vi "Motor_Controller_Tune.vi"(4 "Friction Compensation(F)":bool, 6 "Reinitialize? (F)":bool, 7 "Softload? (T)":bool=TRUE, 8 "error in (no error)":errorcluster, 9 "Mode":T2, 10 "CableTensionRef(N)":dbl[](array[numeric]), 11 "Motor in":refnum<class "MotorControl.lvclass">) -> (0 "error out":errorcluster, 1 "Detailed Voltage":T1, 2 "VoltageCommand":dbl[](array[numeric]) format="%.2f", 3 "Motor out":refnum<class "MotorControl.lvclass">, 5 "PID Gain Idx":i32[](array[numeric]))   [LabVIEW 2015, in "MotorControl.lvclass"]
uses:
  MotorControl.lvclass
  TypeDef/MotorMode.ctl
  MotorControl.lvclass/MotorControl.ctl
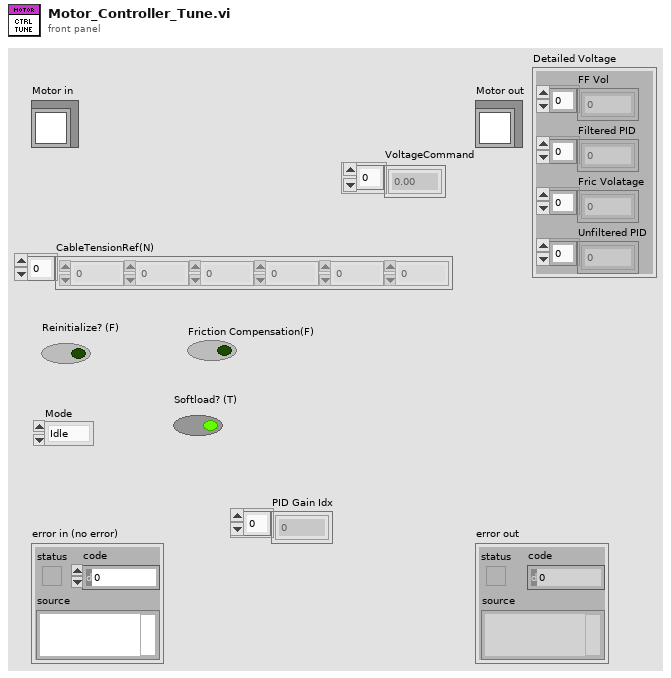
[diagram p1: front panel]
types:
  T1 = cluster{"FF Vol":dbl[], "Filtered PID":dbl[], "Fric Volatage":dbl[], "Unfiltered PID":dbl[]}
  T2 = typedef "MotorControl.lvclass/MotorMode.ctl" = enum16{"Idle", "FF", "PID"}
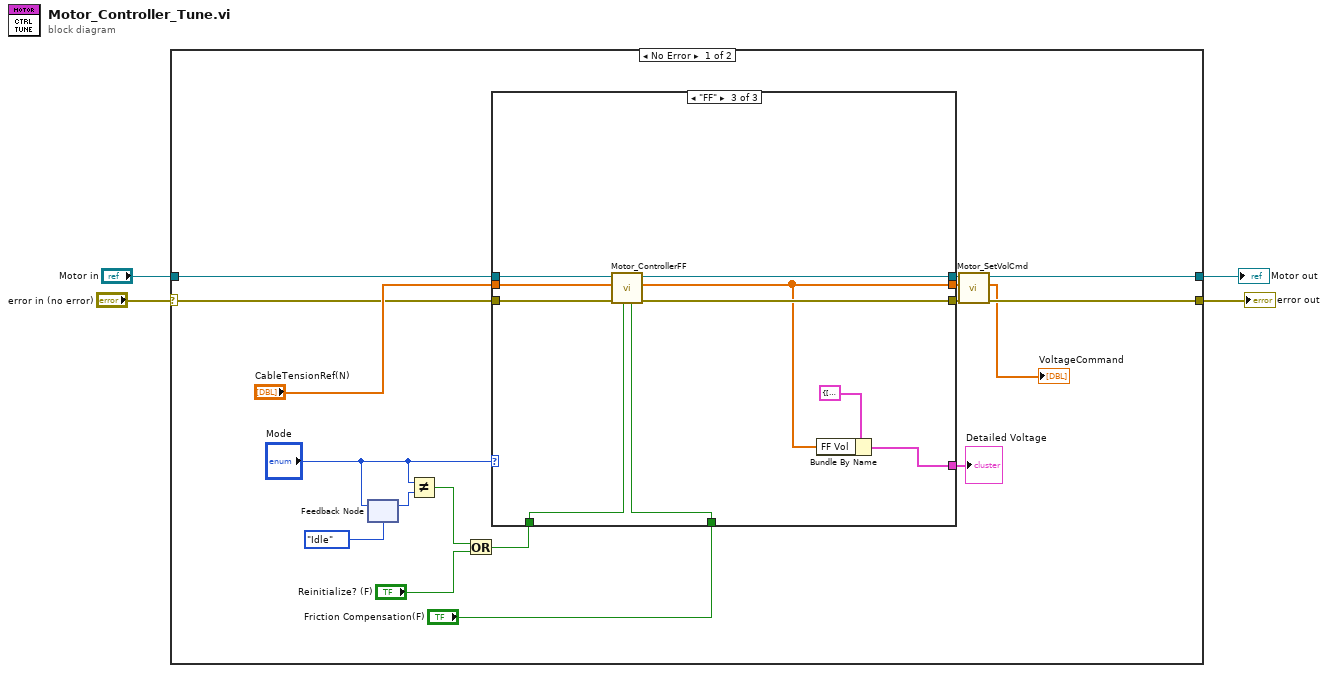
[diagram p0: block diagram]
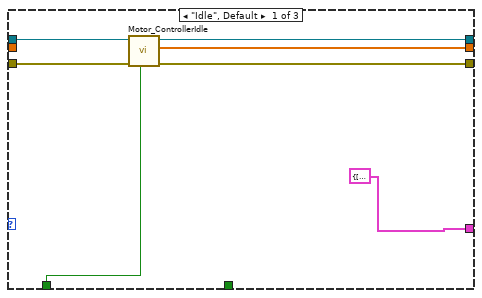
[diagram p2: hidden frame]
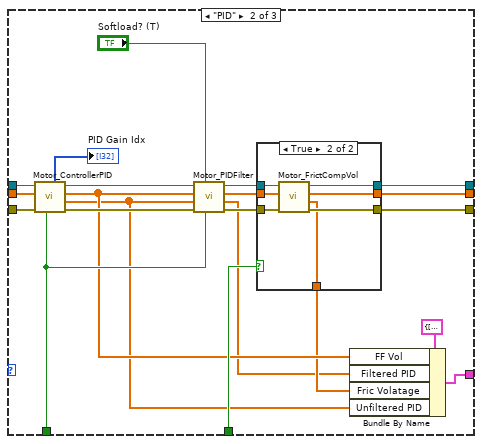
[diagram p3: hidden frame]
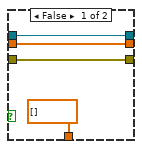
[diagram p4: hidden frame]
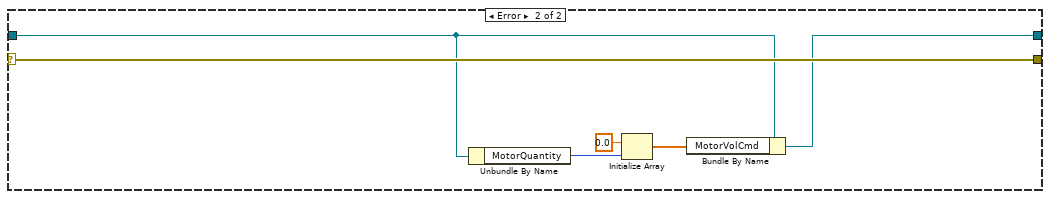
[diagram p5: hidden frame]
diagram:
  n1 = case shown="No Error" "error in (no error)" {
    selector: "error in (no error)" -> [w20 w76]
    tunnel: [w9 w76] -> w3
    tunnel: [w11 w71] -> w1
    tunnel: "Motor in" -> [w19 w72]
    frame No Error {
      n2 = feedback-in #1("Mode") -> ()
      n3 = feedback #1(MotorMode."Idle" ("Mode")) -> (w17:T2)
      n4 = Not Equal?(x="Mode", y=w17) -> (x != y?=w15:bool)
      n5 = Or(x=w15, y="Reinitialize? (F)") -> (x .or. y?=w13:bool)
      n6 = case shown="\"FF\"" "Mode" {
        tunnel: "CableTensionRef(N)" -> [_ w47 w70]
        tunnel: w20 -> [w28 w49 w69]
        tunnel: w19 -> [w27 w48 w68]
        tunnel: w13 -> [w24 w43 w67]
        tunnel: [w25 w39 w66] -> w10
        tunnel: [w26 w40 w65] -> w12
        tunnel: [w23 w36 w63] -> w7
        tunnel: "Friction Compensation(F)" -> [_ w38 w64]
        tunnel: [T1 {"FF Vol"=[], "Filtered PID"=[], "Fric Volatage"=[], "Unfiltered PID"=[]} ("Detailed Voltage") w31 w61] -> w5
        frame "Idle", Default {
          n7 = call "Motor_ControllerIdle.vi"("Reinitialize"=w24, "error in (no error)"=w28, "Motor Control in"=w27) -> ("error out"=w25:errorcluster, "VoltageCommand"=w23:dbl[], "Motor Control out"=w26:refnum<class "MotorControl.lvclass">)  [unwired: 6 in]
        }
        frame "PID" {
          n8 = call "Motor_ControllerPID.vi"("Reinitialize? (F)"=w43, "error in (no error)"=w49, "CableTensionRef(N)"=w47, "Motor in"=w48) -> ("error out"=w45:errorcluster, "PID cmd"=w29:dbl[], "FF cmd"=w34:dbl[], "Motor out"=w46:refnum<class "MotorControl.lvclass">, "PID Gain Idx"=→"PID Gain Idx":i32[])  [unwired: 2 in, 1 out]
          n9 = call "Motor_PIDFilter.vi"("Initialize (F)"=w43, "Softload? (T)"="Softload? (T)", "error in (no error)"=w45, "PID cmd in"=w29, "FF cmd in"=w34, "Motors_New in"=w46) -> ("error out"=w42:errorcluster, "Filtered PID"=w32:dbl[], "Filtered PID + FF"=w37:dbl[], "Motors_New out"=w41:refnum<class "MotorControl.lvclass">)  [unwired: 2 in]
          n10 = case shown="True" w38 {
            tunnel: w42 -> [w52 w60]
            tunnel: w41 -> [w53 w59]
            tunnel: [w53 w58] -> w40
            tunnel: [w52 w57] -> w39
            tunnel: [dbl[] [] ("Fric Volatage") w54] -> w33
            tunnel: w37 -> [w50 w56]
            tunnel: [w50 w55] -> w36
            frame False {
            }
            frame True {
              n11 = call-dynamic "Motor_FrictCompVol.vi"("error in (no error)"=w60, "Input Vol"=w56, "Motor in"=w59) -> ("error out"=w57:errorcluster, "Fric Volatage"=w54:dbl[], "Fric Vol + Input Vol"=w55:dbl[], "Motor out"=w58:refnum<class "MotorControl.lvclass">)  [unwired: 5 in]
            }
          }
          n12 = Bundle By Name(cluster=T1 {"FF Vol"=[], "Filtered PID"=[], "Fric Volatage"=[], "Unfiltered PID"=[]} ("Detailed Voltage"), "FF Vol"=w34, "Filtered PID"=w32, "Fric Volatage"=w33, "Unfiltered PID"=w29) -> (w31:T1)
        }
        frame "FF" {
          n13 = call "Motor_ControllerFF.vi"("Friction Compensation(F)"=w64, "Reinitialize"=w67, "error in (no error)"=w69, "CableTensionRef(N)"=w70, "Motor Control in"=w68) -> ("error out"=w66:errorcluster, "VoltageCommand"=w63:dbl[], "Motor Control out"=w65:refnum<class "MotorControl.lvclass">)  [unwired: 4 in]
          n14 = Bundle By Name(cluster=T1 {"FF Vol"=[], "Filtered PID"=[], "Fric Volatage"=[], "Unfiltered PID"=[]} ("Detailed Voltage"), "FF Vol"=w63) -> (w61:T1)
        }
      }
      "Detailed Voltage" <- w5
      n15 = call "Motor_SetVolCmd.vi"("error in (no error)"=w10, "VolCmd"=w7, "MotorCtrl in"=w12) -> ("error out"=w9:errorcluster, "VolCmdOutput"=→"VoltageCommand":dbl[], "MotorCtrl out"=w11:refnum<class "MotorControl.lvclass">)  [unwired: 6 in]
    }
    frame Error {
      n16 = Unbundle By Name(w72) -> ("MotorQuantity"=w75:i32)
      n17 = Initialize Array(0.0 ("element"), w75) -> (w73:dbl[])
      n18 = Bundle By Name(cluster=w72, "MotorVolCmd"=w73) -> (w71:refnum<class "MotorControl.lvclass">)
    }
  }
  "error out" <- w3
  "Motor out" <- w1
